vi "SeCrTs-Exit FGV.vi"(7 "Enum":enum16{"Init", "Read", "Write"}(ring), 8 "error in":errorcluster, 11 "Exit":bool) -> (0 "error out":errorcluster, 3 "Exit R":bool)   [LabVIEW 2022 SP3]
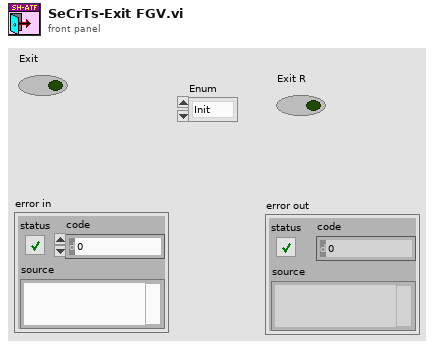
[diagram p1: front panel]
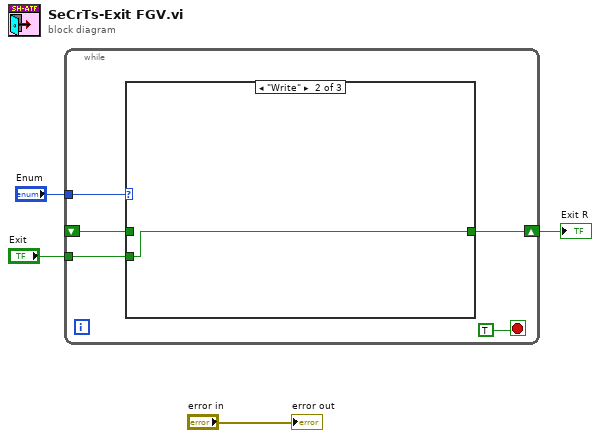
[diagram p0: block diagram]
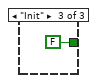
[diagram p3: hidden frame]
diagram:
  n1 = while {
    tunnel: "Enum" -> [w9]
    tunnel: "Exit" -> [w7]
    shift-right: [w6] -> w2
    shift-left: _ -> [w5]
    stop <- TRUE stop-if-true
    n2 = case shown="\"Write\"" w9 {
      tunnel: w7 -> [_ w11 _]
      tunnel: [w10 w11 FALSE ("Exit")] -> w6
      tunnel: w5 -> [w10 _ _]
      frame "Read", Default {
      }
      frame "Write" {
      }
      frame "Init" {
      }
    }
  }
  "Exit R" <- w2
  "error out" <- "error in"
